vi "get dvrs.vi"(11 "Device Data Model in":refnum<class "Standard Data Model.lvclass">) -> (0 "Holding Registers":refnum<data-value>, 1 "Input Registers":refnum<data-value>, 2 "Discrete inputs":refnum<data-value>, 3 "Coils":refnum<data-value>)   [LabVIEW 2021, in "Standard Data Model.lvclass"]
uses:
  Standard Data Model.lvclass
  Standard Data Model.lvclass/Standard Data Model.ctl
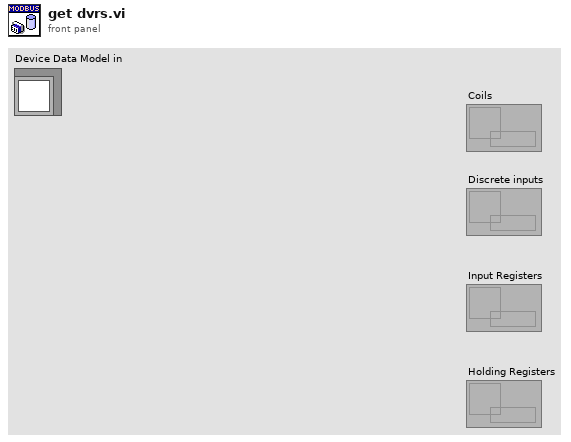
[diagram p1: front panel]
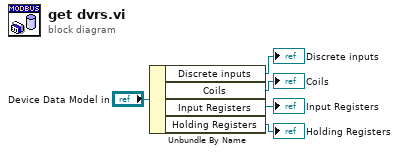
[diagram p0: block diagram]
diagram:
  n1 = Unbundle By Name("Device Data Model in") -> ("Discrete inputs"=→"Discrete inputs":refnum<data-value>, "Coils"=→"Coils":refnum<data-value>, "Input Registers"=→"Input Registers":refnum<data-value>, "Holding Registers"=→"Holding Registers":refnum<data-value>)
